vi "SRV_PM_Timestamp.vi"(12 "Method (Get)":enum16{"Reset", "Get"}(ring)=enum."Get") -> (6 "Timestamp U32":u32, 8 "Timestamp bytes":u8[](array[numeric]))   [LabVIEW 2014]
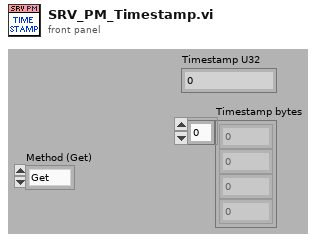
[diagram p1: front panel]
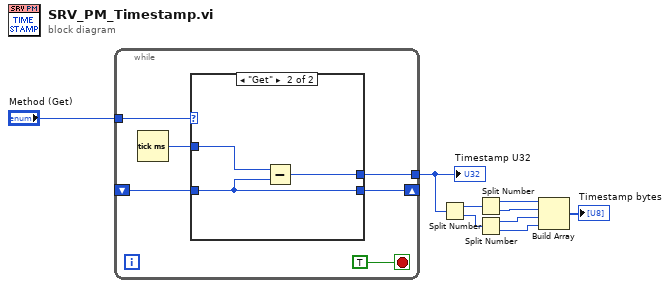
[diagram p0: block diagram]
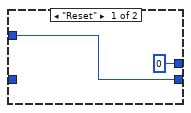
[diagram p2: hidden frame]
diagram:
  n1 = while {
    shift-right: [w10] -> _
    shift-left: _ -> [w14]
    tunnel: "Method (Get)" -> [w13]
    tunnel: [w12] -> w8
    stop <- TRUE stop-if-true
    n2 = Tick Count (ms)() -> (millisecond timer value=w11:u32)
    n3 = case shown="\"Get\"" w13 {
      tunnel: w14 -> [_ w18]
      tunnel: [u32 0 w20] -> w12
      tunnel: w11 -> [w17 w19]
      tunnel: [w17 w18] -> w10
      frame "Reset" {
      }
      frame "Get" {
        n4 = Subtract(x=w19, y=w18) -> (x-y=w20:u32)
      }
    }
  }
  "Timestamp U32" <- w8
  n5 = Split Number(x=w8) -> (hi(x)=w7:u16, lo(x)=w6:u16)
  n6 = Split Number(x=w7) -> (hi(x)=w5:u8, lo(x)=w4:u8)
  n7 = Split Number(x=w6) -> (hi(x)=w3:u8, lo(x)=w2:u8)
  n8 = Build Array(w5, w4, w3, w2) -> (→"Timestamp bytes":u8[])
